vi "未命名 1.vi"() -> ()   [LabVIEW 2019]
panel:
  in  "节点-输出 2":T1(array[cluster])
  out "数据 2":variant
  out "数据":T2
  out "数据字符串":string
  out "值":variant
  in  "节点-输出":T3(array[cluster])
  out "名称":string[](array[string])
  out "数组 2":string[](array[string])
  out "数组":variant[](array[variant])
  in  "簇 7":T4={"ID"=0, "Attribute"="dev", "Action"="", "name"=""} {"ID" format="%02.0f"}
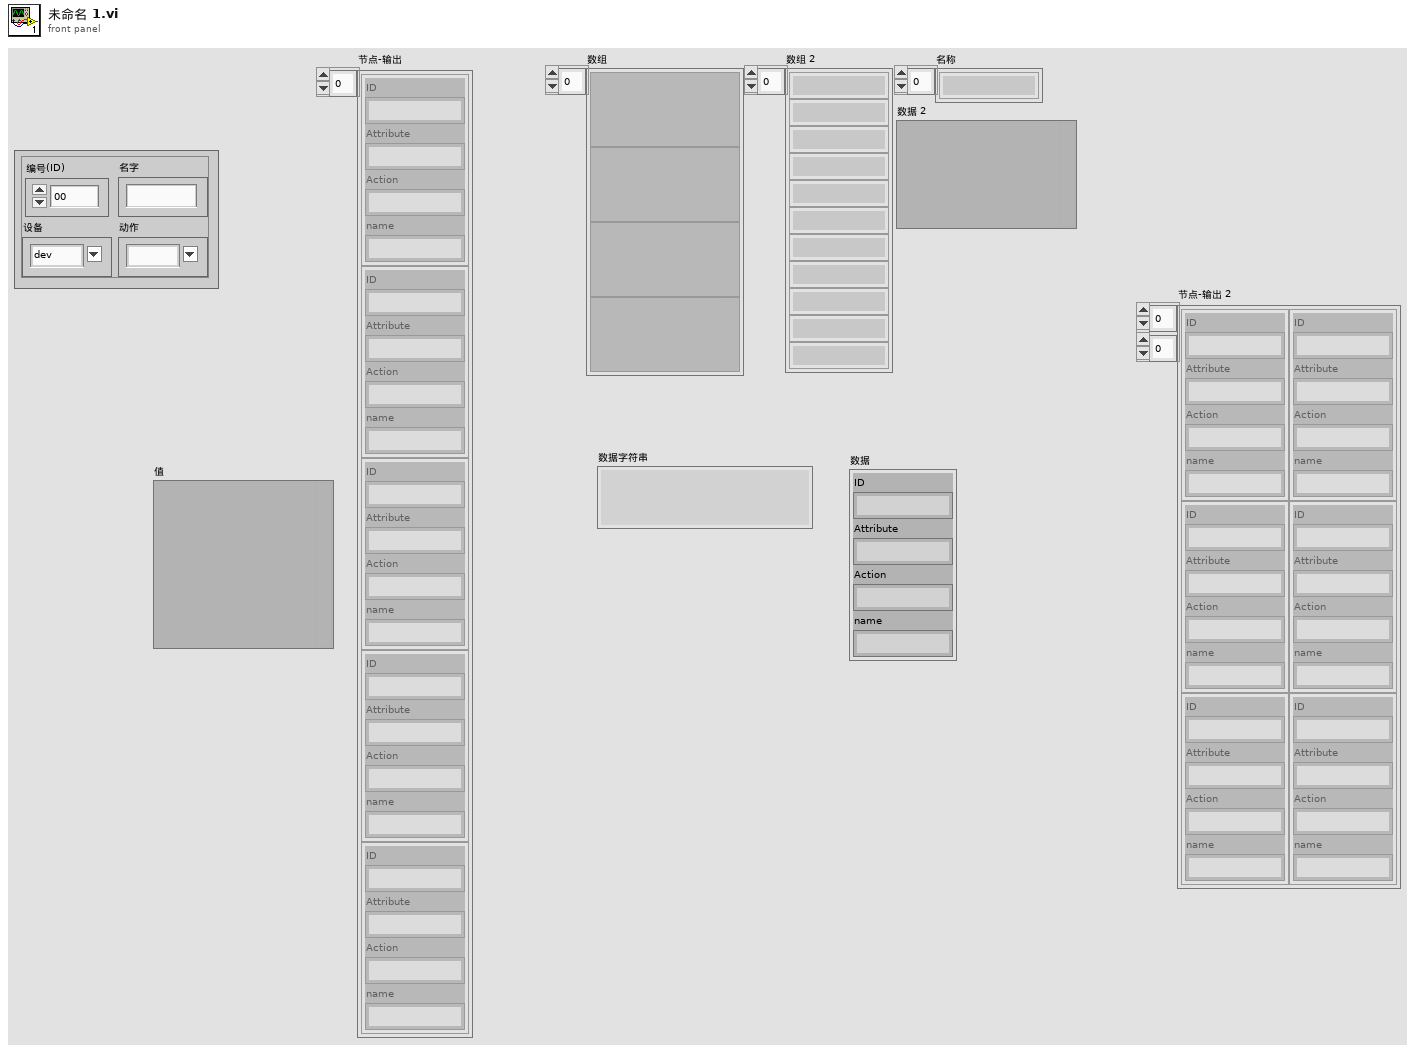
[diagram p1: front panel]
types:
  T1 = cluster{"ID":string, "Attribute":string, "Action":string, "name":string}[][]
  T2 = cluster{"ID":string, "Attribute":string, "Action":string, "name":string}
  T3 = cluster{"ID":string, "Attribute":string, "Action":string, "name":string}[]
  T4 = cluster{"ID":u8, "Attribute":string, "Action":string, "name":string}
  T5 = enum8{"Enabled", "Disabled", "Disabled and Grayed Out"}
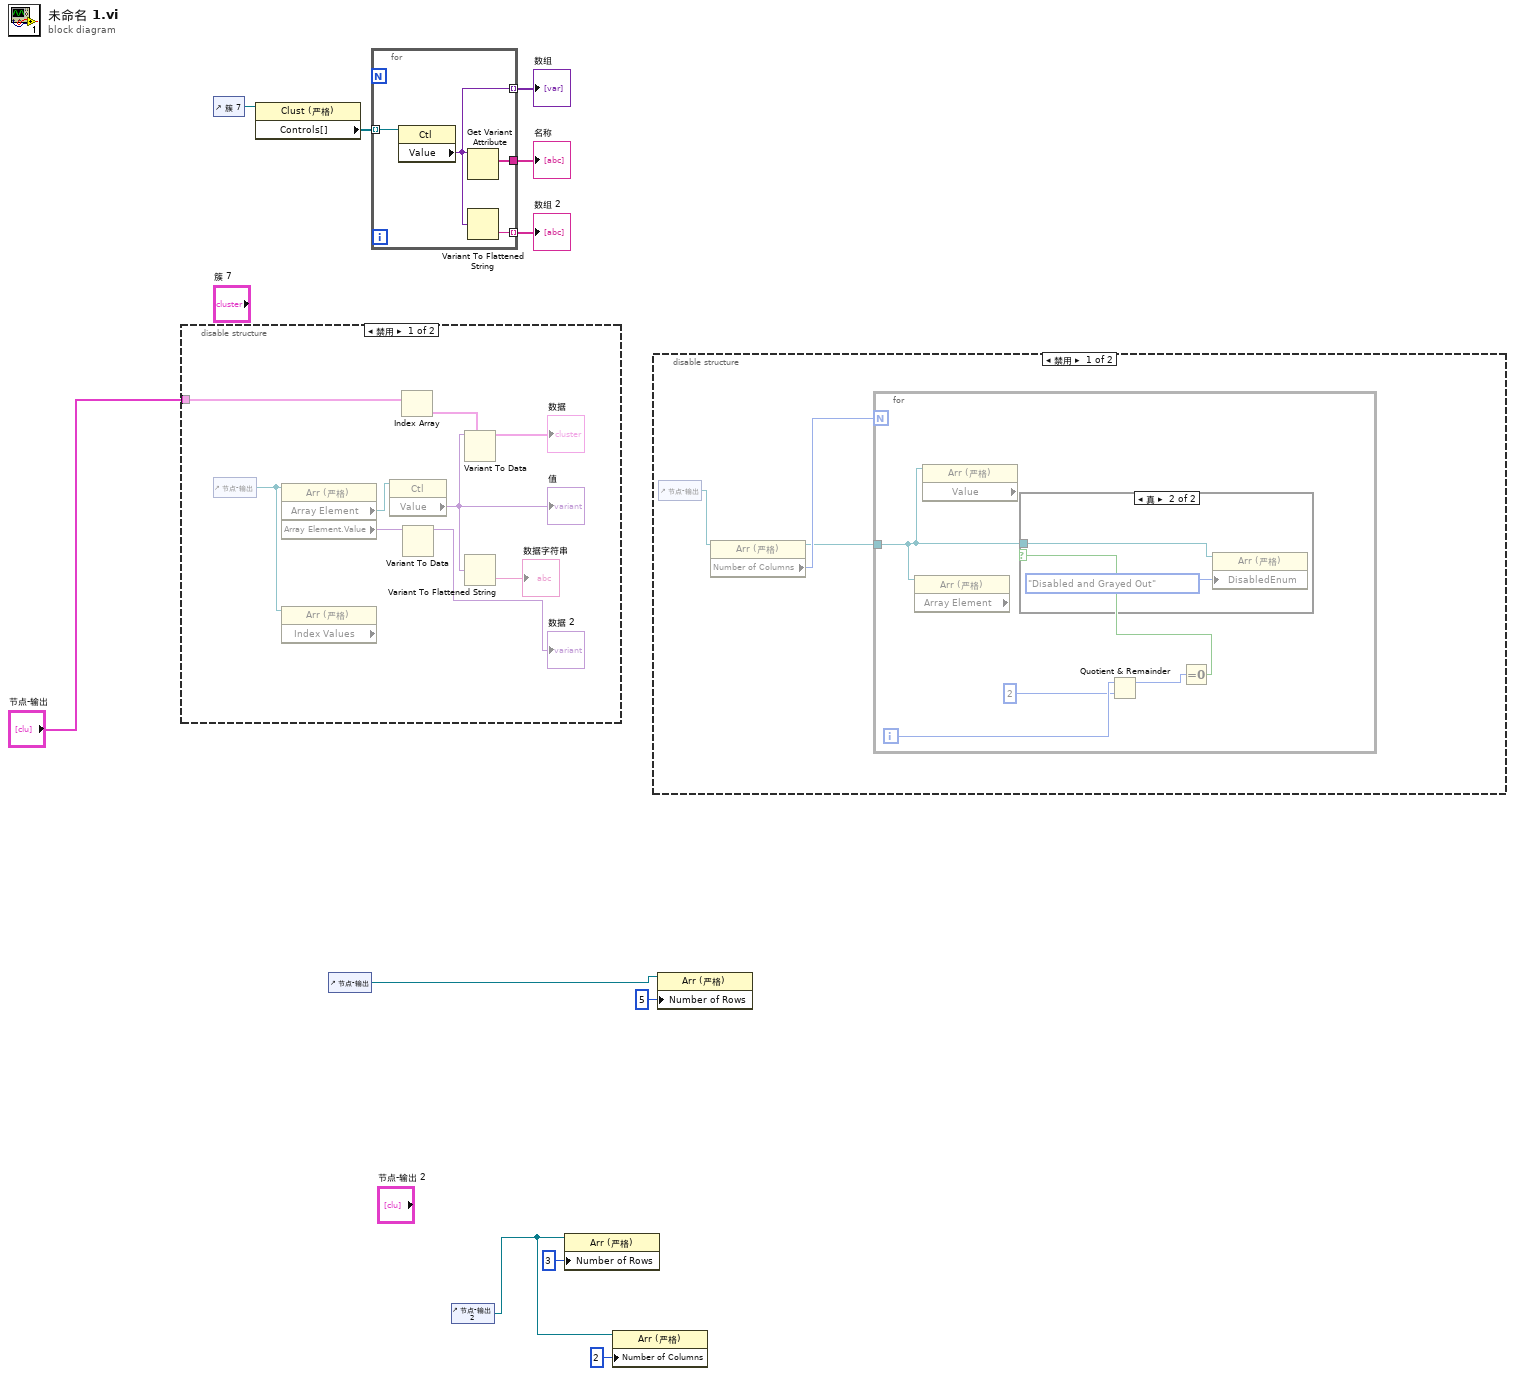
[diagram p0: block diagram]
diagram:
  n1 = disable-structure shown="禁用" {
    disable-tunnel: "节点-输出" -> [w12 _]
    frame Disabled {
      n2 = control-ref of="节点-输出"() -> (w13:refnum<vi>)
      n3 = property class="Arr (严格)"(reference=w13) -> ("Array Element"=w20:refnum<vi>, "Array Element.Value"=w15:variant)  [unwired: 1 in, 2 out]
      n4 = property class="Arr (严格)" props=["Index Values"](reference=w13) -> ()  [unwired: 1 in, 3 out]
      n5 = property class="Ctl"(reference=w20) -> ("Value"=w18:variant)  [unwired: 1 in, 2 out]
      "值" <- w18
      n6 = Index Array(array=w12) -> (element=w17:T2)  [unwired: 1 in]
      n7 = Variant To Data(Variant=w15) -> (data=→"数据 2":variant)  [unwired: 2 in, 1 out]
      n8 = Variant To Data(type=w17, Variant=w18) -> (data=→"数据":T2)  [unwired: 1 in, 1 out]
      n9 = Variant To Flattened String(Variant=w18) -> (data string=→"数据字符串":string)  [unwired: 1 out]
    }
    frame Enabled {
    }
  }
  n10 = control-ref of="簇 7"() -> (w7:refnum<vi>)
  n11 = property class="Clust (严格)"(reference=w7) -> ("Controls[]"=w11:refnum<vi>[])  [unwired: 1 in, 2 out]
  n12 = control-ref of="节点-输出"() -> (w5:refnum<vi>)
  n13 = for {
    tunnel: w11 -> [w24] mode=indexing
    tunnel: [w22] -> w10 mode=indexing
    tunnel: [w23] -> w9 mode=indexing
    tunnel: [w21] -> w8
    n14 = property class="Ctl"(reference=w24) -> ("Value"=w22:variant)  [unwired: 1 in, 2 out]
    n15 = Get Variant Attribute(Variant=w22) -> (names=w21:string[])  [unwired: 3 in, 3 out]
    n16 = Variant To Flattened String(Variant=w22) -> (data string=w23:string)  [unwired: 1 out]
  }
  "数组" <- w10
  "数组 2" <- w9
  "名称" <- w8
  n17 = control-ref of="节点-输出 2"() -> (w2:refnum<vi>)
  n18 = property class="Arr (严格)"(reference=w2, "Number of Rows"=u32 3 ("行数")) -> ()  [unwired: 1 in, 2 out]
  n19 = property class="Arr (严格)"(reference=w2, "Number of Columns"=u32 2 ("列数")) -> ()  [unwired: 1 in, 2 out]
  n20 = disable-structure shown="禁用" {
    frame Disabled {
      n21 = control-ref of="节点-输出"() -> (w27:refnum<vi>)
      n22 = property class="Arr (严格)"(reference=w27) -> (reference out=w25:refnum<vi>, "Number of Columns"=w26:u32)  [unwired: 1 in, 1 out]
      n23 = for {
        N: w26 -> [_]
        tunnel: w25 -> [w28]
        i -> [w32]
        n24 = property class="Arr (严格)" props=["Array Element"](reference=w28) -> ()  [unwired: 1 in, 3 out]
        n25 = property class="Arr (严格)" props=["Value"](reference=w28) -> ()  [unwired: 1 in, 3 out]
        n26 = Quotient & Remainder(x=w32, y=2) -> (x-y*floor(x/y)=w30:i32)  [unwired: 1 out]
        n27 = Equal To 0?(x=w30) -> (x = 0?=w29:bool)
        n28 = case shown="真" w29 {
          tunnel: w28 -> [_ w33]
          frame False {
          }
          frame True {
            n29 = property class="Arr (严格)"(reference=w33, "DisabledEnum"=T5."Disabled and Grayed Out" ("禁用")) -> ()  [unwired: 1 in, 2 out]
          }
        }
      }
    }
    frame Enabled {
    }
  }
  n30 = property class="Arr (严格)"(reference=w5, "Number of Rows"=u32 5 ("行数")) -> ()  [unwired: 1 in, 2 out]
